vi "navX Example v2.vi"() -> ()   [LabVIEW 2015]
uses:
  navX Library v2/_TypeDefs/Flags/Z900_navX_Flags_HardwareRevTypeDef.ctl
  navX Library v2/_TypeDefs/Flags/Z900_navX_Flags_OmnimountConfigTypeDef.ctl
  navX Library v2/_TypeDefs/Z900_navX_SerialStreamTypeDef.ctl
  _NI WPI Serial USB/WPI_SerialPort_USB.ctl
  <vilib>/Rock Robotics/SystemInterfaces/i2clib/i2c_bus.ctl
  <vilib>/Rock Robotics/SystemInterfaces/spilib/spi_bus.ctl
  navX Library v2/_TypeDefs/Flags/Z900_navX_Flags_OpStatusTypeDef.ctl
  navX Library v2/_TypeDefs/Flags/Z900_navX_Flags_CalibrationStatusTypeDef.ctl
  <vilib>/Platform/TimedLoop/XDataNode/timing_clust.ctl
  <vilib>/Platform/TimedLoop/XDataNode/nitl_modes.ctl
  <vilib>/Platform/TimedLoop/XDataNode/wakeup.ctl
  navX Library v2/_Util/Decode Protocol/Z900_navX_Util_DecodeProtocol_UInt16.vi
  navX Library v2/_Util/Decode Protocol/Z900_navX_Util_DecodeProtocol_UInt32.vi
  navX Library v2/_Util/Decode Protocol/Z900_navX_Util_DecodeProtocol_SignedHundredths.vi
  navX Library v2/_Util/Decode Protocol/Z900_navX_Util_DecodeProtocol_SignedRatio.vi
  navX Library v2/_Util/Decode Protocol/Z900_navX_Util_DecodeProtocol_UnsignedHundredths.vi
  navX Library v2/_Util/Decode Protocol/Z900_navX_Util_DecodeProtocol_1616.vi
  navX Library v2/_Util/Decode Protocol/Z900_navX_Util_DecodeProtocol_SignedThousandths.vi
  navX Library v2/_Util/Decode Protocol/Z900_navX_Util_DecodeProtocol_Int16.vi
  navX Library v2/_Util/Z900_navX_Util_LittleEndian_to_BigEndian.vi
  navX Library v2/_Util/Decode Protocol/Z900_navX_Util_DecodeProtocol_Int32.vi
  navX Library v2/Device/_Open/Z900_navX_Open_Serial.vi
  navX Library v2/Device/_Open/Z900_navX_Open_I2C.vi
  navX Library v2/Device/_Open/Z900_navX_Open_SPI.vi
  navX Library v2/Device/_Internal/Z900_navX_Internal_Get.vi
  <vilib>/platform/TimedLoop/XDataNode/XDataNode.xnode
  navX Library v2/navX Library v2.lvlib
  _NI WPI Serial USB/_NI WPI Serial USB.lvlib
  <vilib>/Platform/TimedLoop/XDataNode/XDNodeRunTimeDep.lvlib
panel:
  in  "Zero Displacement":bool
  out "Status":T3 {"OP Status" items=["INITIALIZING", "SELFTEST_IN_PROGRESS", "ERROR", "IMU_AUTOCAL_IN_PROGRESS", "NORMAL"]; "Calibration Status" items=["IMU_CAL_STATE_MASK"=3, "IMU_CAL_STATE_INPROGRESS"=0, "IMU_CAL_STATE_ACCUMULATE"=1, "IMU_CAL_STATE_COMPLETE"=2]}
  out "Connected":bool
  out "ERROR!":bool
  in  "Enable Logs":bool
  in  "Clear Log":bool
  out "Internal Error Log":errorcluster[](array[cluster])
  out "Log Size":i32
  in  "Interface Control":enum32{"Serial", "I2C", "SPI"}(tab)=enum."SPI"
  in  "Serial Port":T4=enum."MXP TTL"
  in  "Update Stream Type":bool
  in  "Stream Type":T5=enum."AHRS"
  in  "I2C Bus":T6=enum."I2C MXP"
  in  "SPI Bus":T7=enum."SPI MXP"
  in  "Clock Rate (Hz)":dbl=2000000.0 format="%_6f"
  in  "Zero Yaw":bool
  out "Raw Values":T8
  out "Quaternion":T9
  out "Linear Acceleration":T10
  out "Displacement":T11
  out "Offsets":T12
  out "Timestamp":u32
  out "MPUTemp":dbl(slide) scale=20.0..50.0
  in  "Update Rate":u8=50 min=4 max=60
  out "Board Information":T15 {"Board"."Hardware Revision" items=["navX-MXP"=33, "navX-Micro"=40]; "Omnimount Config" items=["DEFAULT", "X_UP", "X_DOWN", "Y_UP", "Y_DOWN", "Z_UP", "Z_DOWN"]}
  out "YRPHfH":T16
  in  "stop":bool
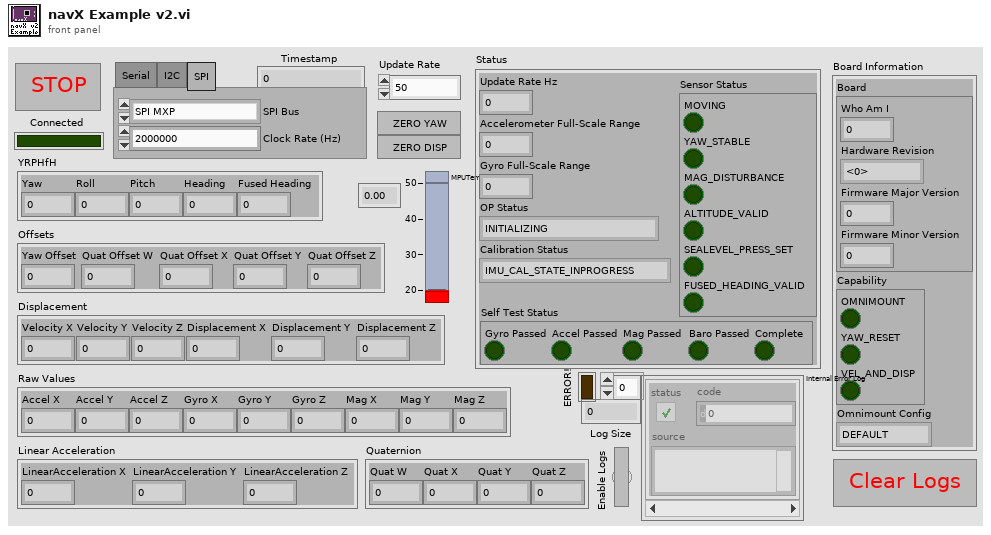
[diagram p1: front panel]
types:
  T1 = typedef "navX Library v2.lvlib/Z900_navX_Flags_OpStatusTypeDef.ctl" = u8
  T2 = typedef "navX Library v2.lvlib/Z900_navX_Flags_CalibrationStatusTypeDef.ctl" = u8
  T3 = cluster{"Update Rate Hz":u8, "Accelerometer Full-Scale Range":u8, "Gyro Full-Scale Range":u16, "OP Status":T1, "Calibration Status":T2, "Sensor Status":cluster{"MOVING":bool, "YAW_STABLE":bool, "MAG_DISTURBANCE":bool, "ALTITUDE_VALID":bool, "SEALEVEL_PRESS_SET":bool, "FUSED_HEADING_VALID":bool}, "Self Test Status":cluster{"Gyro Passed":bool, "Accel Passed":bool, "Mag Passed":bool, "Baro Passed":bool, "Complete":bool}}
  T4 = typedef "_NI WPI Serial USB.lvlib/WPI_SerialPort_USB.ctl" = enum16{"Onboard RS-232", "MXP TTL", "USB"}
  T5 = typedef "navX Library v2.lvlib/Z900_navX_SerialStreamTypeDef.ctl" = enum16{"YRPH", "Quaterinons", "Gyro/Raw", "AHRS", "AHRSAndPositioning"}
  T6 = typedef "i2c_bus.ctl" = enum16{"I2C On-Board", "I2C MXP", "Invalid"}
  T7 = typedef "spi_bus.ctl" = enum16{"SPI On-Board, CS0", "SPI On-Board, CS1", "SPI On-Board, CS2", "SPI On-Board, CS3", "SPI MXP", "Invalid"}
  T8 = cluster{"Accel X":dbl, "Accel Y":dbl, "Accel Z":dbl, "Gyro X":dbl, "Gyro Y":dbl, "Gyro Z":dbl, "Mag X":dbl, "Mag Y":dbl, "Mag Z":dbl}
  T9 = cluster{"Quat W":dbl, "Quat X":dbl, "Quat Y":dbl, "Quat Z":dbl}
  T10 = cluster{"LinearAcceleration X":dbl, "LinearAcceleration Y":dbl, "LinearAcceleration Z":dbl}
  T11 = cluster{"Velocity X":dbl, "Velocity Y":dbl, "Velocity Z":dbl, "Displacement X":dbl, "Displacement Y":dbl, "Displacement Z":dbl}
  T12 = cluster{"Yaw Offset":dbl, "Quat Offset W":dbl, "Quat Offset X":dbl, "Quat Offset Y":dbl, "Quat Offset Z":dbl}
  T13 = typedef "navX Library v2.lvlib/Z900_navX_Flags_HardwareRevTypeDef.ctl" = u8
  T14 = typedef "navX Library v2.lvlib/Z900_navX_Flags_OmnimountConfigTypeDef.ctl" = u8
  T15 = cluster{"Board":cluster{"Who Am I":u8, "Hardware Revision":T13, "Firmware Major Version":u8, "Firmware Minor Version":u8}, "Capability":cluster{"OMNIMOUNT":bool, "YAW_RESET":bool, "VEL_AND_DISP":bool}, "Omnimount Config":T14}
  T16 = cluster{"Yaw":dbl, "Roll":dbl, "Pitch":dbl, "Heading":dbl, "Fused Heading":dbl}
  T17 = cluster{"Interface Control":enum32{"Serial", "I2C", "SPI"}, "Serial Port":T4, "I2C Bus":T6, "SPI Bus":T7, u8, "Clock Rate (Hz)":dbl}
  T18 = typedef "XDNodeRunTimeDep.lvlib/timing_clust.ctl" = cluster{"Expected End [f-1]":u64, "Actual End [f-1]":u64, "Finished Late? [f-1]":bool, "Expected End [i-1]":u64, "Actual End [i-1]":u64, "Finished Late? [i-1]":bool, "Expected Start [i]":u64, "Actual Start [i]":u64, "Expected Start [f]":u64, "Actual Start [f]":u64, "Source Name":string, "Structure Name":string, "Period":i64, "Deadline":i64, "Offset":i64, "Start":i64, "Priority":i32, "Timeout":i32, "Mode":T19, "Wakeup Reason":T20, "Error":errorcluster, "Source Type":string, "Secondary Source Type":string, "Global End Time":u64, "Global Start Time":u64, "Frame Duration":u64, "Iteration Duration":u64, "Assigned CPU":i32, "I/O Scan Engine Mode":u32}
  T19 = typedef "XDNodeRunTimeDep.lvlib/nitl_modes.ctl" = enum32{"No Change", "Process missed periods, maintain original phase", "Discard missed periods, maintain original phase", "Process missed periods, ignore original phase", "Discard missed periods, ignore original phase"}
  T20 = typedef "XDNodeRunTimeDep.lvlib/wakeup.ctl" = enum32{"Normal", "Aborted", "Asynchronous wakeup", "Timing source error", "Timed loop error", "Timeout"}
  T21 = cluster{"Interface Control":bool, "Serial Port":bool, "I2C Bus":bool, "SPI Bus":bool, bool, "Clock Rate (Hz)":bool}
  T22 = typedef "navX Library v2.lvlib/Z900_navX_DeviceTypeDef.ctl" = cluster{"Interface":cluster{"Protocol":T23, "Update Rate (4Hz-100Hz)":u8, "navX Open TypeDef":variant}, "Notify Packet":refnum<notifier>, "Loop VI Refnum":refnum<vi>, "Ready to Close Occurrence Refnum":refnum<k4>}
  T23 = typedef "navX Library v2.lvlib/Z900_navX_ProtocolTypeDef.ctl" = enum16{"SERIAL", "I2C", "SPI"}
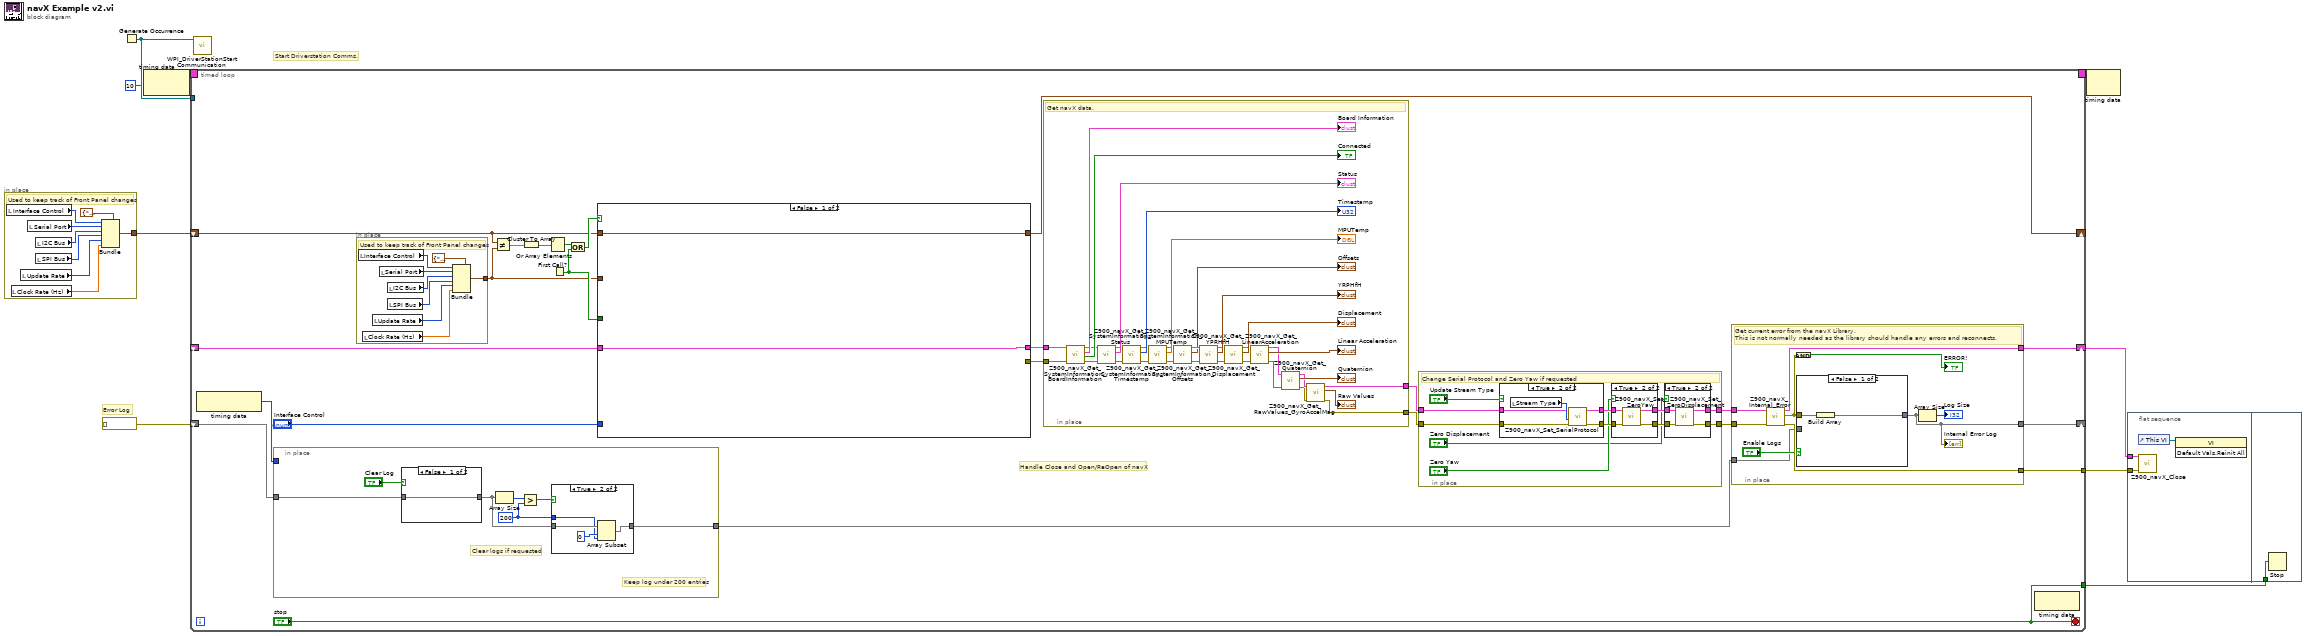
[diagram p0: block diagram]
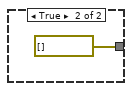
[diagram p3: hidden frame]
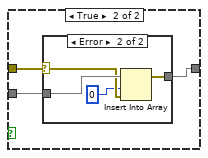
[diagram p4: hidden frame]
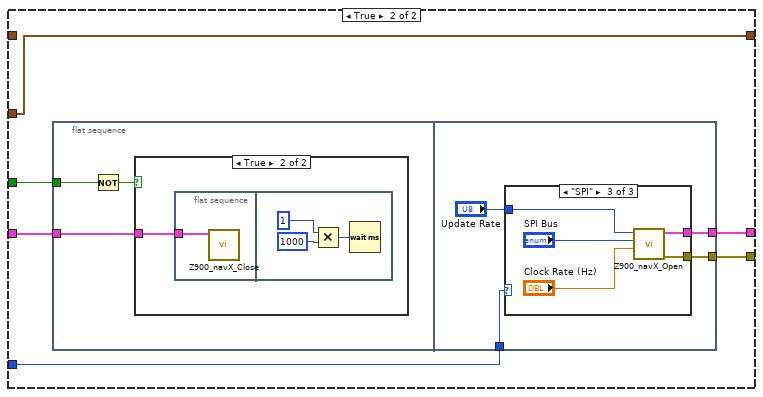
[diagram p9: hidden frame]
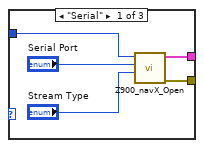
[diagram p11: hidden frame]
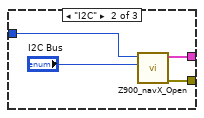
[diagram p12: hidden frame]
diagram:
  # "Start Driverstation Comms."
  # "Error Log"
  n1 = in-place {
    in-place-border: [w16] -> w6
    # "Used to keep track of Front Panel changes"
    n2 = local read "Interface Control"() -> (w15:enum32{"Serial", "I2C", "SPI"})
    n3 = local read "Clock Rate (Hz)"() -> (w10:dbl)
    n4 = local read "Update Rate"() -> (w11:u8)
    n5 = local read "Serial Port"() -> (w14:T4)
    n6 = local read "I2C Bus"() -> (w13:T6)
    n7 = local read "SPI Bus"() -> (w12:T7)
    n8 = Bundle(cluster=T17 {"Interface Control"=enum."Serial", "Serial Port"=enum."Onboard RS-232", "I2C Bus"=enum."I2C On-Board", "SPI Bus"=enum."SPI On-Board, CS0", 0, "Clock Rate (Hz)"=0.0} ("output cluster"), "Interface Control"=w15, "Serial Port"=w14, "I2C Bus"=w13, "SPI Bus"=w12, w11, "Clock Rate (Hz)"=w10) -> (w16:T17)
  }
  n9 = Generate Occurrence() -> (w5:refnum<k4>)
  n10 = node-c288(i64 10 ("Period")) -> (w3:T18)
  n11 = timed-loop {
    shift-right: [w36] -> w9
    shift-left: _ -> [w34]
    shift-right: [w35] -> _
    shift-left: errorcluster[] [] -> [w22]
    tunnel: [w19] -> w7
    shift-right: [w25] -> _
    shift-left: w6 -> [w24]
    tunnel: w5 -> [_]
    tunnel: ["stop"] -> w4
    timing: w3 -> [_]
    timing-out: [_] -> w2
    stop <- "stop" stop-if-true
    # "Handle Close and Open/ReOpen of navX"
    n12 = node-c288() -> (w18:i64)  [unwired: 1 in]
    n13 = in-place {
      in-place-border: w22 -> [w58]
      in-place-border: [w54] -> w21
      in-place-border: w18 -> [_]
      w53 = 200 ("y")
      # "Clear logs if requested"
      # "Keep log under 200 entries"
      n14 = case shown="False" "Clear Log" {
        tunnel: [w64 errorcluster[] []] -> w52
        tunnel: w58 -> [w64 _]
        frame False {
        }
        frame True {
        }
      }
      n15 = Array Size(array=w52) -> (size(s)=w57:i32)
      n16 = Greater?(x=w57, y=w53) -> (0:w55:bool)
      n17 = case shown="True" w55 {
        tunnel: [w59 w60] -> w54
        tunnel: w52 -> [w59 w63]
        tunnel: w53 -> [_ w61]
        frame False {
        }
        frame True {
          n18 = Array Subset(array=w63, index=0, length=w61) -> (w60:errorcluster[])
        }
      }
    }
    n19 = in-place {
      in-place-border: [w50] -> w20
      # "Used to keep track of Front Panel changes"
      n20 = local read "Interface Control"() -> (w49:enum32{"Serial", "I2C", "SPI"})
      n21 = local read "Clock Rate (Hz)"() -> (w44:dbl)
      n22 = local read "Update Rate"() -> (w45:u8)
      n23 = local read "Serial Port"() -> (w48:T4)
      n24 = local read "I2C Bus"() -> (w47:T6)
      n25 = local read "SPI Bus"() -> (w46:T7)
      n26 = Bundle(cluster=T17 {"Interface Control"=enum."Serial", "Serial Port"=enum."Onboard RS-232", "I2C Bus"=enum."I2C On-Board", "SPI Bus"=enum."SPI On-Board, CS0", 0, "Clock Rate (Hz)"=0.0} ("output cluster"), "Interface Control"=w49, "Serial Port"=w48, "I2C Bus"=w47, "SPI Bus"=w46, w45, "Clock Rate (Hz)"=w44) -> (w50:T17)
    }
    n27 = Not Equal?(x=w24, y=w20) -> (x != y?=w28:T21)
    n28 = Cluster To Array(cluster=w28) -> (array=w27:bool[])
    n29 = Or Array Elements(Boolean array=w27) -> (logical OR=w26:bool)
    n30 = First Call?() -> (First Call?: T/F=w30:bool)
    n31 = Or(x=w26, y=w30) -> (x .or. y?=w31:bool)
    n32 = case shown="False" w31 {
      tunnel: w34 -> [w150 w156]
      tunnel: [w150 w151] -> w33
      tunnel: [_ w155] -> w32
      tunnel: "Interface Control" -> [_ w154]
      tunnel: w30 -> [_ w153]
      tunnel: w20 -> [_ w152]
      tunnel: [w149 w152] -> w25
      tunnel: w24 -> [w149 _]
      frame False {
      }
      frame True {
        n33 = flat-sequence {
          tunnel: w153 -> [w157]
          tunnel: w156 -> [w158]
          tunnel: [w167] -> w151
          tunnel: [w166] -> w155
          tunnel: w154 -> [w165]
          frame #0 {
            n34 = Not(x=w157) -> (.not. x?=w159:bool)
            n35 = case shown="True" w159 {
              tunnel: w158 -> [_ w160]
              frame False {
              }
              frame True {
                n36 = flat-sequence {
                  tunnel: w160 -> [w161]
                  frame #0 {
                    n37 = call "Z900_navX_Close.vi"("navX Device"=w161) -> ()  [unwired: 10 in, 1 out]
                  }
                  frame #1 {
                    n38 = Multiply(x=u32 1, y=u32 1000 ("x")) -> (x*y=w163:u32)
                    n39 = Wait (ms)(milliseconds to wait=w163) -> ()  [unwired: 1 out]
                  }
                }
              }
            }
          }
          frame #1 {
            n40 = case shown="\"SPI\"" w165 {
              tunnel: [w171 w175 w181] -> w167
              tunnel: [w170 w174 w180] -> w166
              tunnel: "Update Rate" -> [w169 w177 w179]
              frame "Serial" {
                n41 = call-poly "Z900_navX_Open.vi"("Stream Type"="Stream Type", "Serial Port"="Serial Port", "Update Rate (4Hz-60Hz)"=w169) -> ("error out"=w170:errorcluster, "navX Device"=w171:T22)  [unwired: 7 in]
              }
              frame "I2C" {
                n42 = call-poly "Z900_navX_Open.vi"("I2C Bus"="I2C Bus", "Update Rate (4Hz-60Hz)"=w177) -> ("error out"=w174:errorcluster, "navX Device"=w175:T22)  [unwired: 8 in]
              }
              frame "SPI" {
                n43 = call-poly "Z900_navX_Open.vi"("Clock Rate (Hz)"="Clock Rate (Hz)", "SPI Bus"="SPI Bus", "Update Rate (4Hz-60Hz)"=w179) -> ("error out"=w180:errorcluster, "navX Device"=w181:T22)  [unwired: 7 in]
              }
            }
          }
        }
      }
    }
    n44 = in-place {
      in-place-border: [w136] -> w40
      in-place-border: [w135] -> w39
      in-place-border: w33 -> [w134]
      in-place-border: w32 -> [w133]
      # "Get navX data."
      n45 = call "Z900_navX_Get_SystemInformation_BoardInformation.vi"("error in (no error)"=w133, "navX Device"=w134) -> ("error out"=w129:errorcluster, "Connected"=→"Connected":bool, "Board Information"=→"Board Information":T15, "navX Device"=w128:T22)  [unwired: 6 in]
      n46 = call "Z900_navX_Get_SystemInformation_Status.vi"("error in (no error)"=w129, "navX Device"=w128) -> ("error out"=w127:errorcluster, "Status"=→"Status":T3, "navX Device"=w126:T22)  [unwired: 6 in, 1 out]
      n47 = call "Z900_navX_Get_SystemInformation_Timestamp.vi"("error in (no error)"=w127, "navX Device"=w126) -> ("error out"=w124:errorcluster, "Timestamp"=→"Timestamp":u32, "navX Device"=w125:T22)  [unwired: 6 in, 1 out]
      n48 = call "Z900_navX_Get_SystemInformation_MPUTemp.vi"("error in (no error)"=w124, "navX Device"=w125) -> ("error out"=w122:errorcluster, "MPUTemp"=→"MPUTemp":dbl, "navX Device"=w123:T22)  [unwired: 6 in, 1 out]
      n49 = call "Z900_navX_Get_SystemInformation_Offsets.vi"("error in (no error)"=w122, "navX Device"=w123) -> ("error out"=w145:errorcluster, "Offsets"=→"Offsets":T12, "navX Device"=w146:T22)  [unwired: 6 in, 1 out]
      n50 = call "Z900_navX_Get_YPRHfH.vi"("error in (no error)"=w145, "navX Device"=w146) -> ("error out"=w143:errorcluster, "YRPHfH"=→"YRPHfH":T16, "navX Device"=w144:T22)  [unwired: 6 in, 1 out]
      n51 = call "Z900_navX_Get_Displacement.vi"("error in (no error)"=w143, "navX Device"=w144) -> ("error out"=w120:errorcluster, "Displacement"=→"Displacement":T11, "navX Device"=w121:T22)  [unwired: 6 in, 1 out]
      n52 = call "Z900_navX_Get_LinearAcceleration.vi"("error in (no error)"=w120, "navX Device"=w121) -> ("error out"=w118:errorcluster, "Linear Acceleration"=→"Linear Acceleration":T10, "navX Device"=w119:T22)  [unwired: 6 in, 1 out]
      n53 = call "Z900_navX_Get_Quaternion.vi"("error in (no error)"=w118, "navX Device"=w119) -> ("error out"=w116:errorcluster, "Quaternion"=→"Quaternion":T9, "navX Device"=w117:T22)  [unwired: 6 in, 1 out]
      n54 = call "Z900_navX_Get_RawValues_GyroAccelMag.vi"("error in (no error)"=w116, "navX Device"=w117) -> ("error out"=w135:errorcluster, "Raw Values"=→"Raw Values":T8, "navX Device"=w136:T22)  [unwired: 6 in, 1 out]
    }
    n55 = in-place {
      in-place-border: w40 -> [w96]
      in-place-border: w39 -> [w95]
      in-place-border: [w88] -> w38
      in-place-border: [w87] -> w37
      # "Change Serial Protocol and Zero Yaw if requested"
      n56 = case shown="True" "Update Stream Type" {
        tunnel: w96 -> [w110 w114]
        tunnel: [w110 w113] -> w94
        tunnel: w95 -> [w109 w112]
        tunnel: [w109 w111] -> w93
        frame False {
        }
        frame True {
          n57 = local read "Stream Type"() -> (w115:T5)
          n58 = call "Z900_navX_Set_SerialProtocol.vi"("error in (no error)"=w112, "Stream Type"=w115, "navX Device"=w114) -> ("error out"=w111:errorcluster, "navX Device"=w113:T22)  [unwired: 7 in]
        }
      }
      n59 = case shown="True" "Zero Yaw" {
        tunnel: w94 -> [w104 w108]
        tunnel: [w104 w107] -> w90
        tunnel: w93 -> [w103 w106]
        tunnel: [w103 w105] -> w89
        frame False {
        }
        frame True {
          n60 = call "Z900_navX_Set_ZeroYaw.vi"("error in (no error)"=w106, "navX Device"=w108) -> ("error out"=w105:errorcluster, "navX Device"=w107:T22)  [unwired: 8 in]
        }
      }
      n61 = case shown="True" "Zero Displacement" {
        tunnel: w90 -> [w98 w102]
        tunnel: [w98 w101] -> w88
        tunnel: w89 -> [w97 w100]
        tunnel: [w97 w99] -> w87
        frame False {
        }
        frame True {
          n62 = call "Z900_navX_Set_ZeroDisplacement.vi"("error in (no error)"=w100, "navX Device"=w102) -> ("error out"=w99:errorcluster, "navX Device"=w101:T22)  [unwired: 8 in]
        }
      }
    }
    n63 = in-place {
      in-place-border: w38 -> [w75]
      in-place-border: w37 -> [w74]
      in-place-border: [w73] -> w36
      in-place-border: [w72] -> w35
      in-place-border: [w70] -> w19
      in-place-border: w21 -> [w68]
      # "Get current error from the navX Library.\nThis is not normally needed as the library should handle any errors and reconnects."
      n64 = call "Z900_navX_Internal_Error.vi"("error in (no error)"=w74, "navX Device"=w75) -> ("error out"=w70:errorcluster, "Internal error out"=w67:errorcluster, "navX Device"=w73:T22)  [unwired: 7 in]
      n65 = Compound Arithmetic op=AND(w67) -> (→"ERROR!":bool)
      n66 = case shown="False" "Enable Logs" {
        tunnel: w67 -> [w77 w80]
        tunnel: [w76 w79] -> w72
        tunnel: w68 -> [_ w78]
        frame False {
          n67 = Build Array(w77) -> (w76:errorcluster[])
        }
        frame True {
          n68 = case shown="Error" w80 {
            selector: w80 -> [_ w84]
            tunnel: [w81 w82] -> w79
            tunnel: w78 -> [w81 w85]
            frame No Error {
            }
            frame Error {
              n69 = Insert Into Array(array=w85, index=0, new element=w84) -> (w82:errorcluster[])
            }
          }
        }
      }
      "Internal Error Log" <- w72
      n70 = Array Size(array=w72) -> (size(s)=→"Log Size":i32)
    }
    n71 = node-c288() -> ()  [unwired: 1 in, 1 out]
  }
  n72 = call <vilib>:"WPI_DriverStationStart Communication.vi"("occurrence"=w5) -> ()  [unwired: 11 in]
  n73 = node-c288(w2) -> ()  [unwired: 1 out]
  n74 = flat-sequence {
    tunnel: w9 -> [w185]
    tunnel: w7 -> [w184]
    tunnel: w4 -> [w186]
    frame #0 {
      n75 = control-ref of="This VI"() -> (w183:refnum<vi>)
      n76 = call "Z900_navX_Close.vi"("error in (no error)"=w184, "navX Device"=w185) -> ()  [unwired: 9 in, 1 out]
      n77 = invoke class="VI" method="Default Vals.Reinit All"(reference=w183) -> ()  [unwired: 2 in, 3 out]
    }
    frame #1 {
      n78 = Stop(stop? (T)=w186) -> ()
    }
  }
